vi "iPSread.vi"(8 "error in (no error)":errorcluster, 10 "iPSreadCtrl":T1=enum."Switch Heater Temp", 11 "VISA resource name":refnum<visa-resource-name>) -> (0 "error out":errorcluster, 1 "read buffer":string, 2 "number":dbl, 3 "VISA resource name out":refnum<visa-resource-name>)   [LabVIEW 2021]
uses:
  controls/iPSreadCtrl.ctl
  <vilib>/regexp/Match Regular Expression.xnode
panel:
  out "after match":string
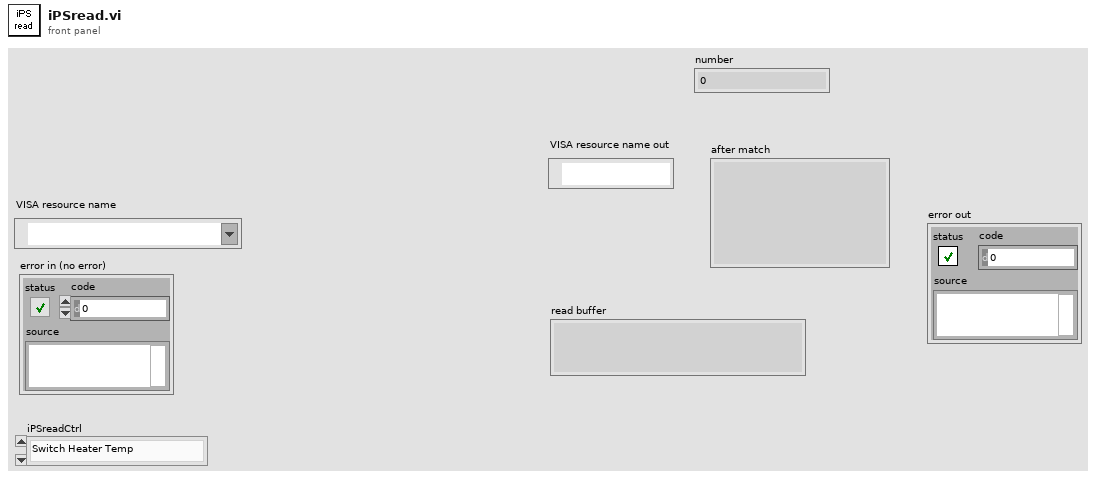
[diagram p1: front panel]
types:
  T1 = typedef "iPSreadCtrl.ctl" = enum16{"OutputField", "MagnetField", "Switch Heater Temp", "Field Rate", "Magnet Temp", "OutputVoltage"}
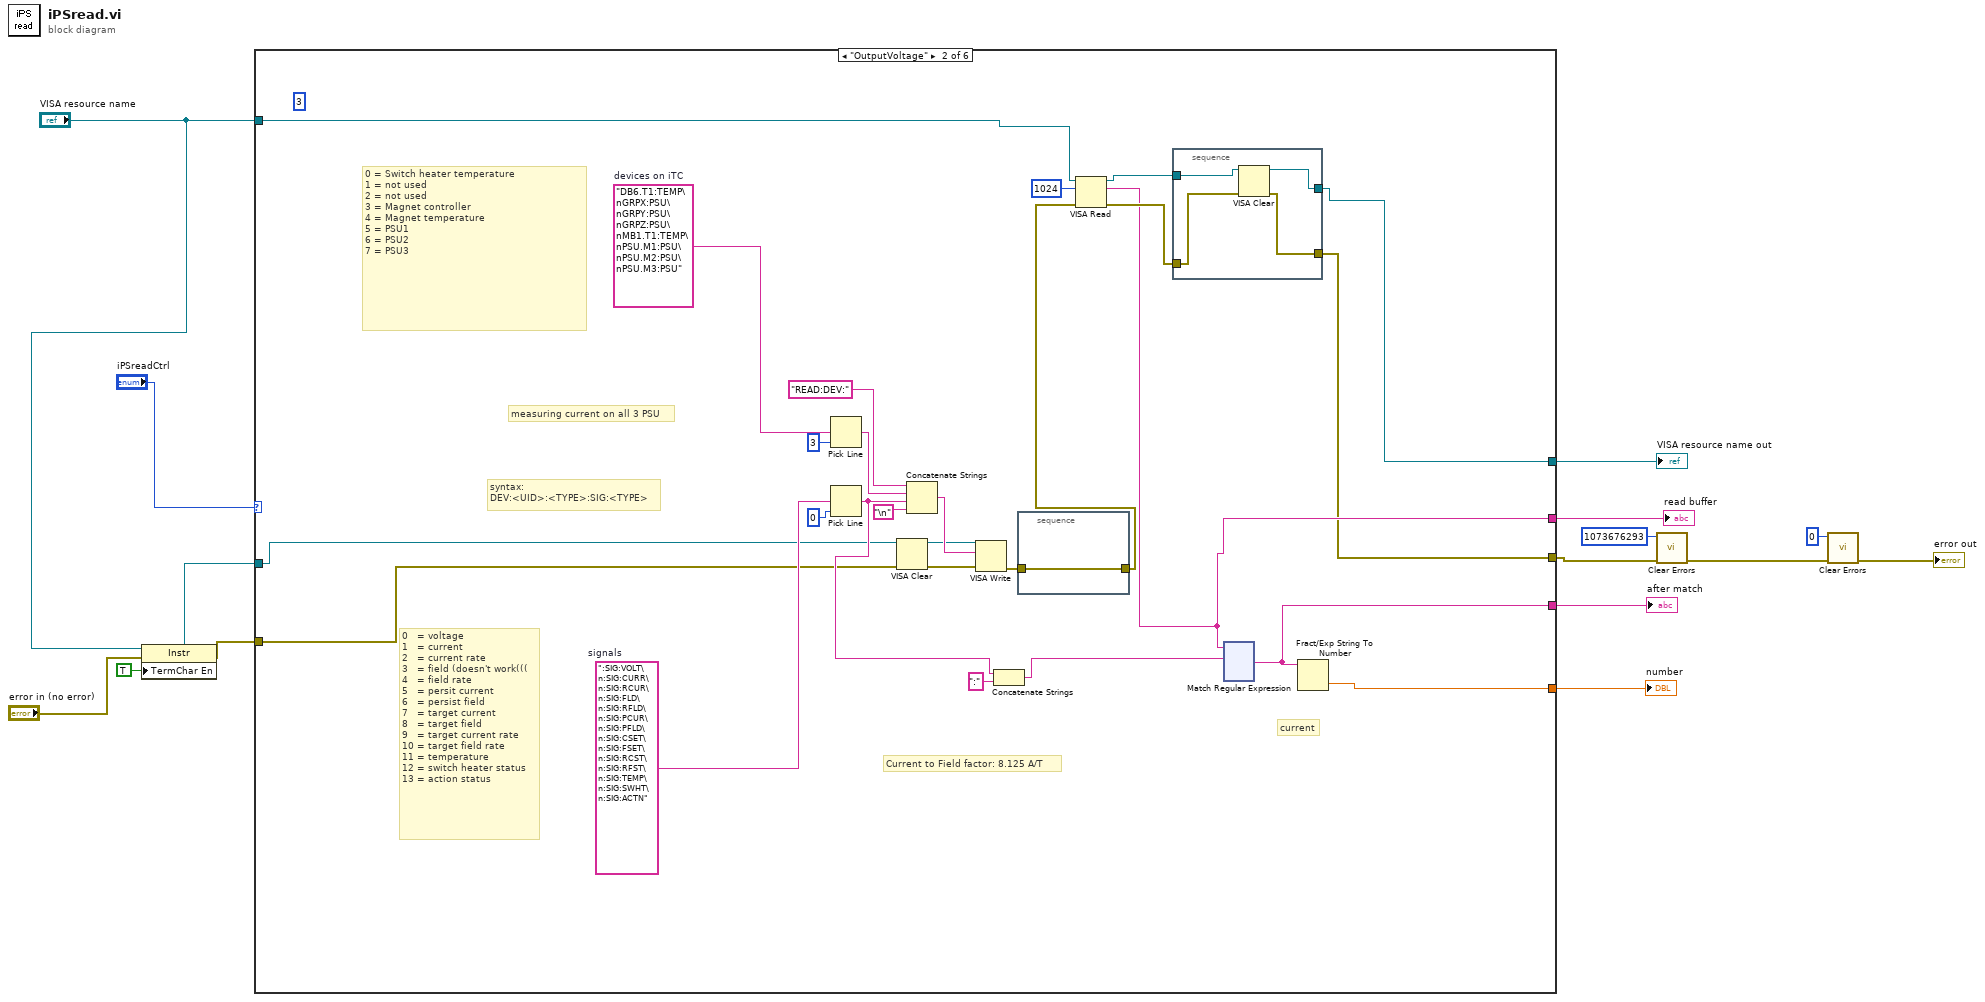
[diagram p0: block diagram]
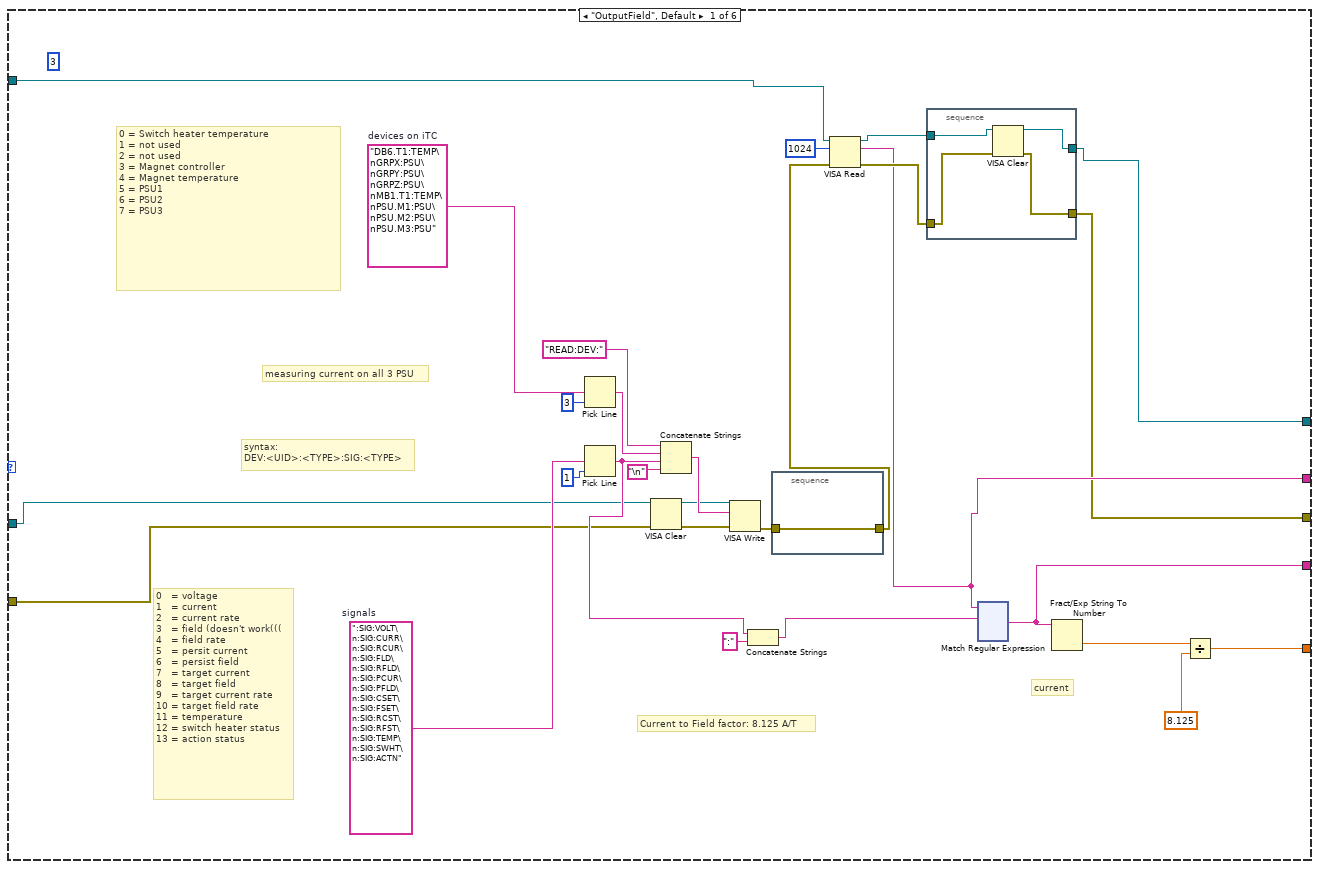
[diagram p2: hidden frame]
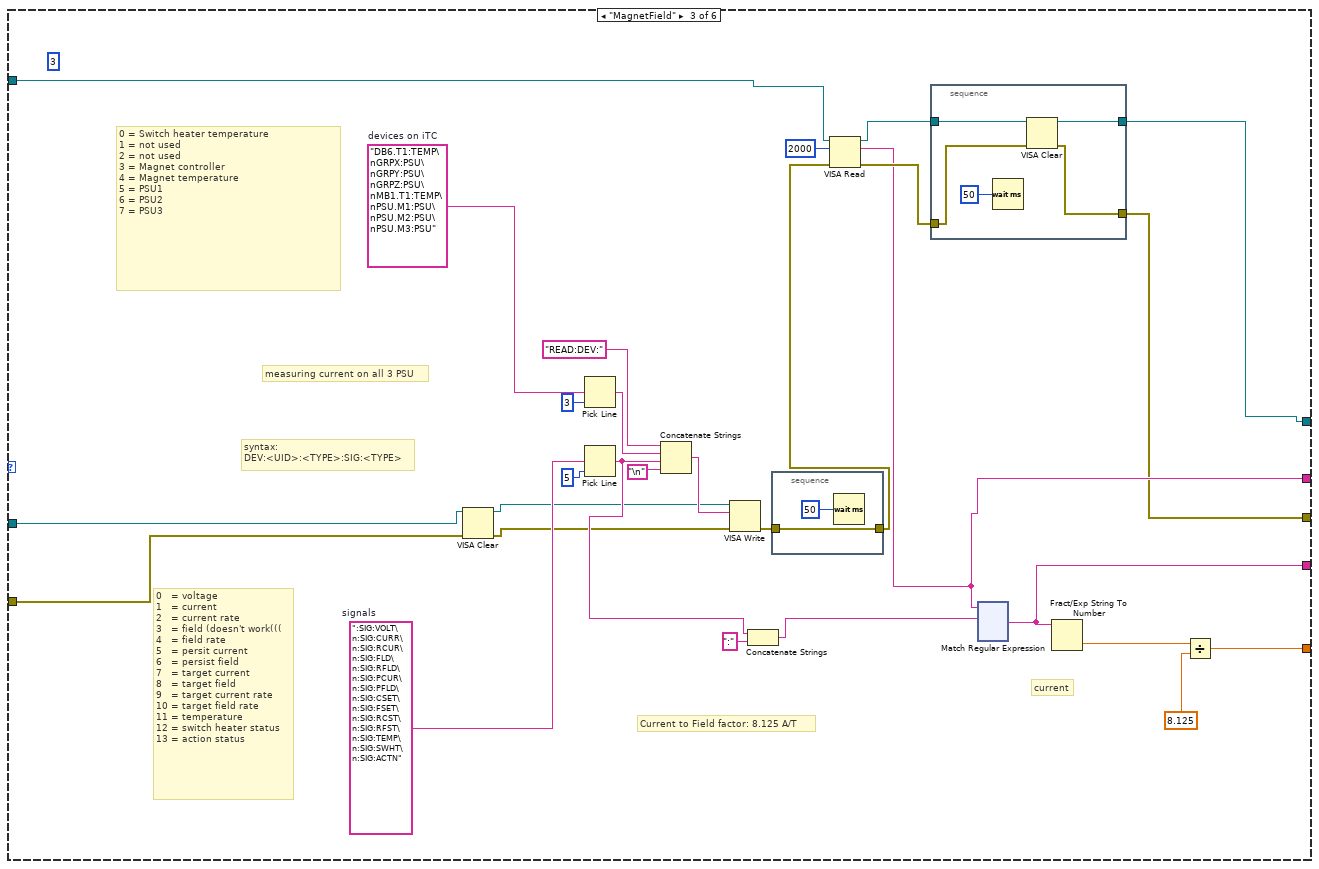
[diagram p3: hidden frame]
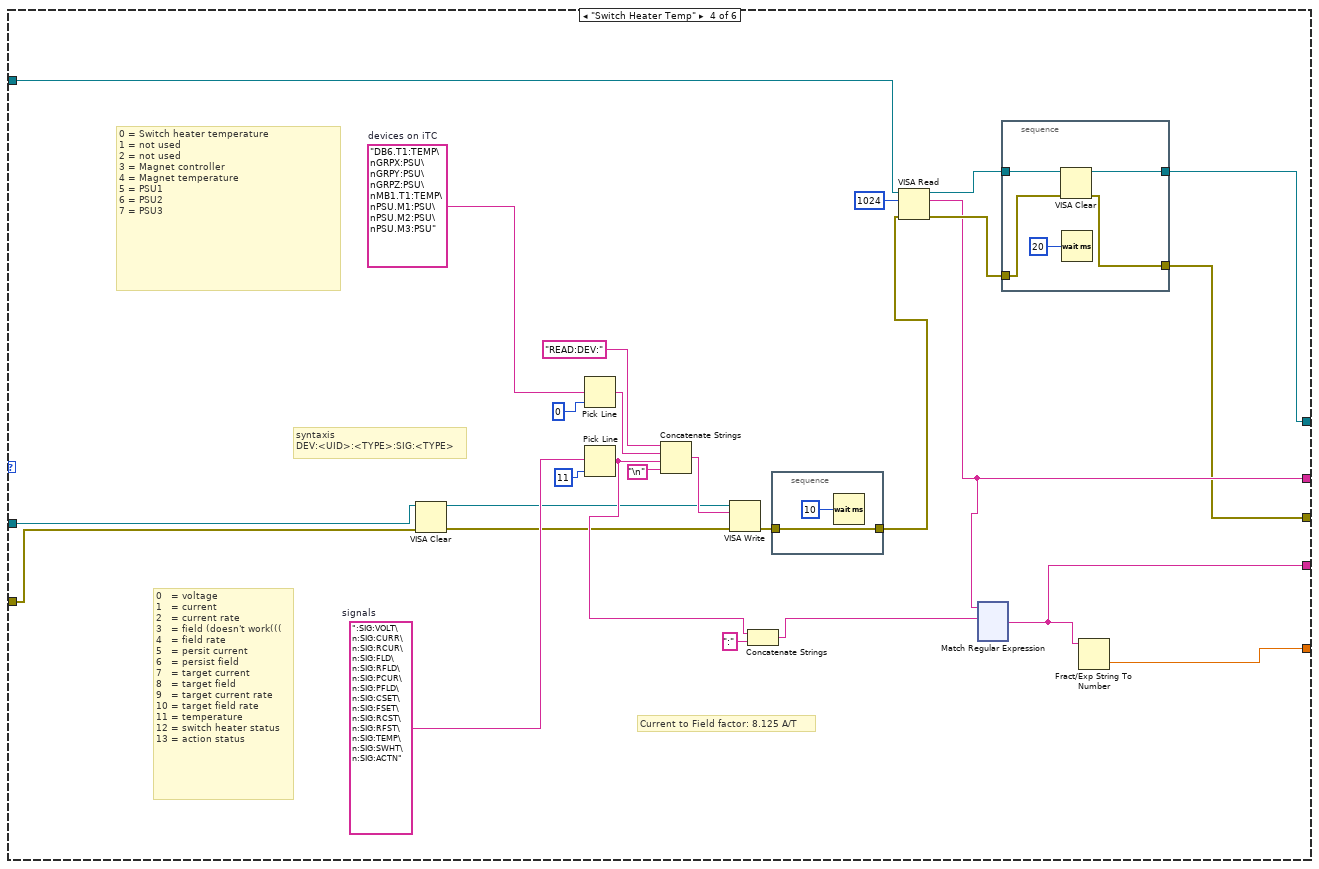
[diagram p4: hidden frame]
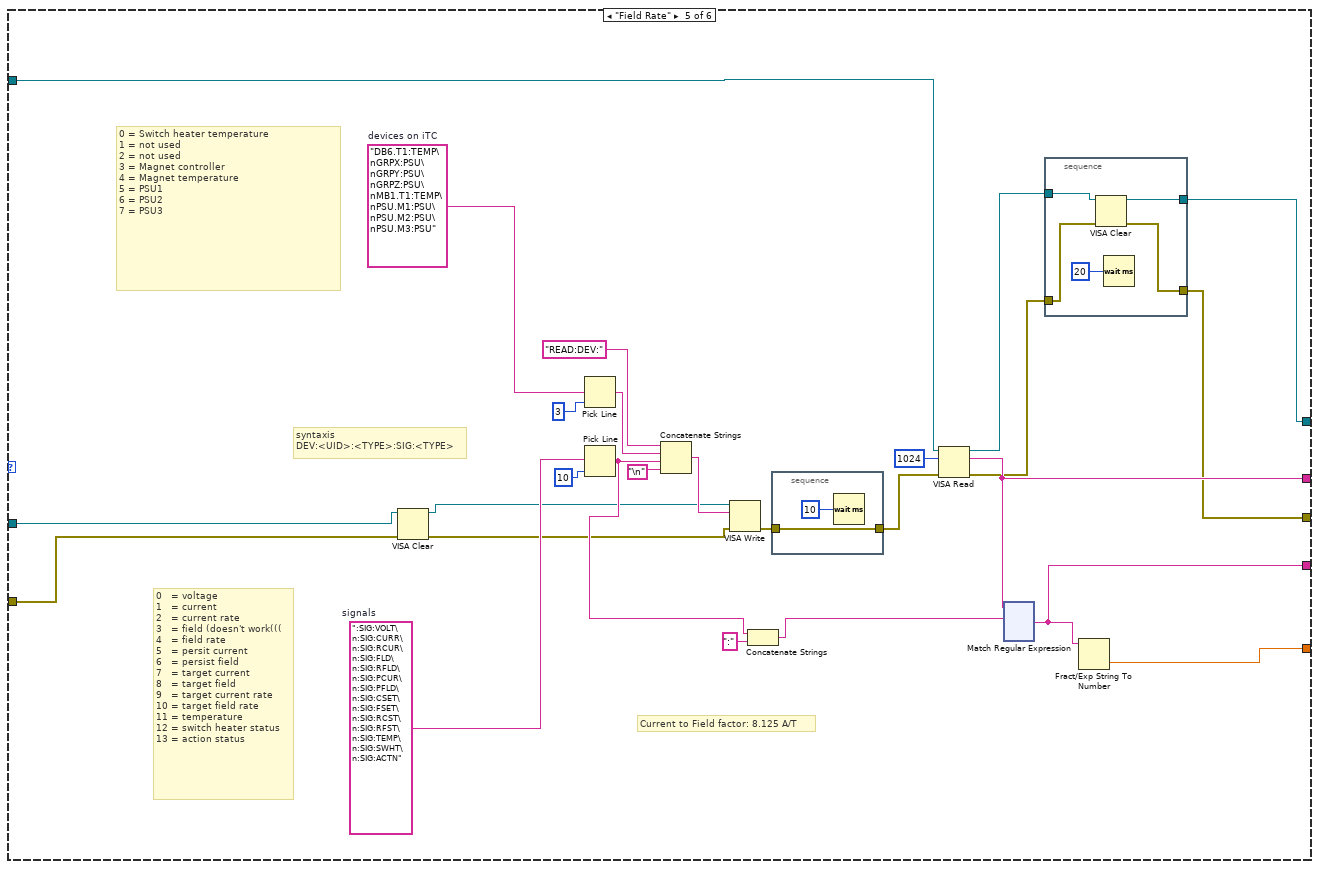
[diagram p5: hidden frame]
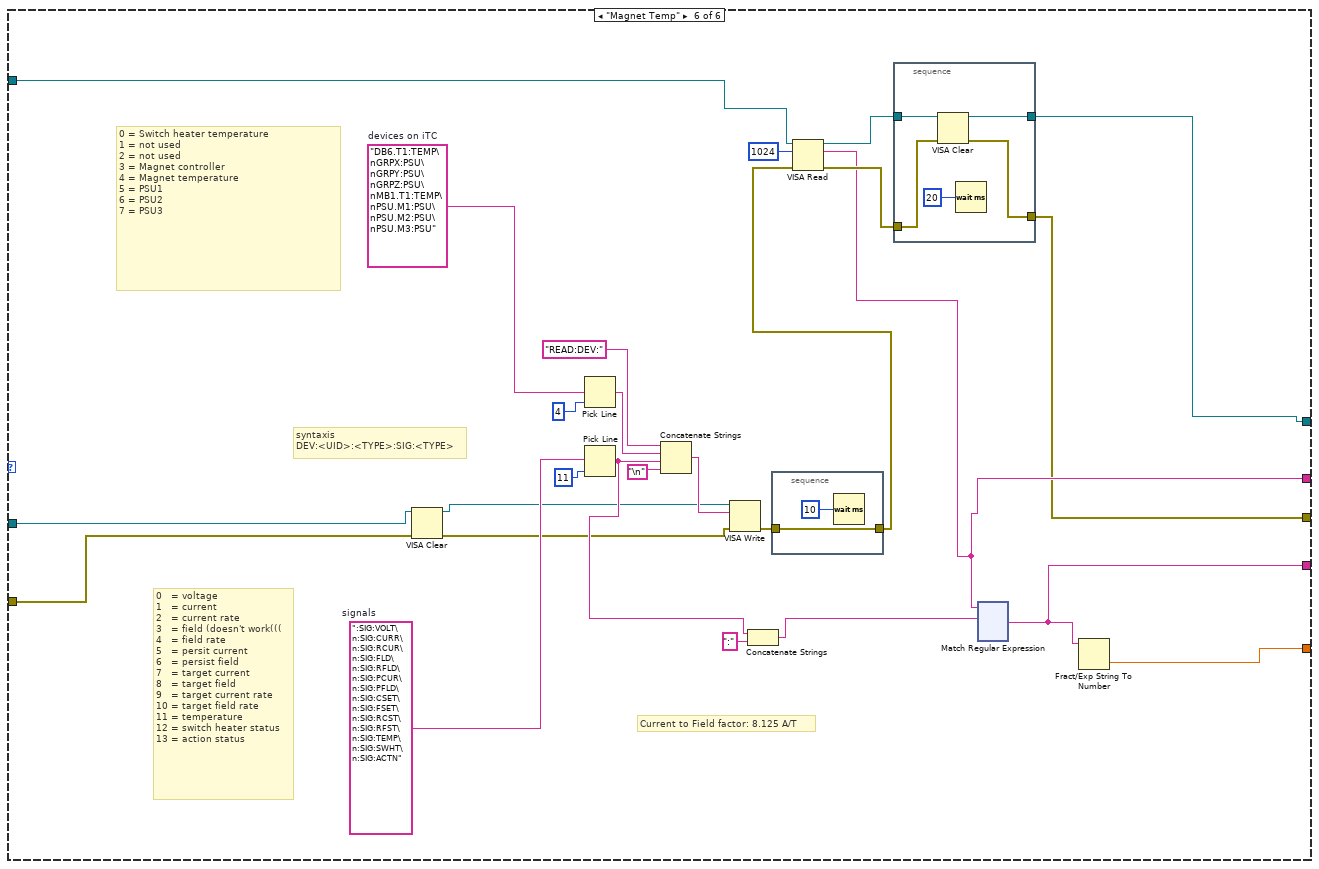
[diagram p6: hidden frame]
diagram:
  n1 = property class="Instr"(reference="VISA resource name", error in="error in (no error)", "TermChar En"=TRUE ("Message Based Settings:Termination Character Enable")) -> (reference out=w9:refnum<visa-resource-name>, error out=w7:errorcluster)
  n2 = case shown="\"OutputVoltage\"" "iPSreadCtrl" {
    tunnel: "VISA resource name" -> [w22 w173 w320 w472 w622 w775]
    tunnel: [w23 w174 w321 w473 w623 w772] -> w5
    tunnel: [w16 w167 w314 w467 w616 w767] -> w15
    tunnel: [w24 w175 w322 w475 w626 w773] -> w14
    tunnel: [w43 w191 w341 w481 w631 w781] -> w13
    tunnel: [w41 w166 w339 w480 w630 w780] -> w12
    tunnel: w7 -> [w20 w171 w316 w468 w620 w768]
    tunnel: w9 -> [w21 w172 w317 w469 w621 w769]
    frame "OutputField", Default {
      w35 = ":SIG:VOLT\n:SIG:CURR\n:SIG:RCUR\n:SIG:FLD\n:SIG:RFLD\n:SIG:PCUR\n:SIG:PFLD\n:SIG:CSET\n:SIG:FSET\n:SIG:RCST\n:SIG:RFST\n:SIG:TEMP\n:SIG:SWHT\n:SIG:ACTN"  # signals
      w40 = "DB6.T1:TEMP\nGRPX:PSU\nGRPY:PSU\nGRPZ:PSU\nMB1.T1:TEMP\nPSU.M1:PSU\nPSU.M2:PSU\nPSU.M3:PSU"  # devices on iTC
      (unwired) 3
      # "current"
      # "measuring current on all 3 PSU"
      # "Current to Field factor: 8.125 A/T"
      # "0 = Switch heater temperature\n1 = not used\n2 = not used\n3 = Magnet controller \n4 = Magnet temperature\n5 = PSU1 \n6 = PSU2\n7 = PSU3"
      # "0   = voltage\n1   = current\n2   = current rate\n3   = field (doesn't work(((\n4   = field rate\n5   = persit current\n6   = persist field\n7   = target current\n8   = target field\n9   = target current rate\n10 = target field rate \n11 = temperature\n12 = switch heater status\n13 = action status"
      # "syntax:\nDEV:<UID>:<TYPE>:SIG:<TYPE>"
      n3 = Pick Line(multi-line string=w40, line index=3) -> (output string=w37:string)  [unwired: 1 in]
      n4 = Pick Line(multi-line string=w35, line index=1) -> (output string=w33:string)  [unwired: 1 in]
      n5 = VISA Clear(VISA resource name=w21, error in (no error)=w20) -> (VISA resource name out=w19:refnum<visa-resource-name>, error out=w18:errorcluster)
      n6 = Concatenate Strings("READ:DEV:" ("write buffer"), w37, w33, "\n") -> (w31:string)
      n7 = VISA Write(VISA resource name=w19, write buffer=w31, error in (no error)=w18) -> (error out=w39:errorcluster)  [unwired: 2 out]
      n8 = Concatenate Strings(w33, ":" ("string")) -> (w32:string)
      n9 = stacked-sequence {
        tunnel: w39 -> [w165]
        tunnel: [w165] -> w25
        frame #0 {
        }
      }
      n10 = VISA Read(VISA resource name=w22, byte count=u32 1024, error in (no error)=w25) -> (VISA resource name out=w17:refnum<visa-resource-name>, read buffer=w24:string, error out=w26:errorcluster)  [unwired: 1 out]
      n11 = stacked-sequence {
        tunnel: [w46] -> w23
        tunnel: w26 -> [w45]
        tunnel: w17 -> [w44]
        tunnel: [w47] -> w16
        frame #0 {
          n12 = VISA Clear(VISA resource name=w44, error in (no error)=w45) -> (VISA resource name out=w47:refnum<visa-resource-name>, error out=w46:errorcluster)
        }
      }
      n13 = xnode "Match Regular Expression"("input string"=w24, "regular expression"=w32) -> ("after match"=w43:string)  [unwired: 4 in, 4 out]
      n14 = Fract/Exp String To Number(string=w43) -> (number=w28:dbl)  [unwired: 3 in, 1 out]
      n15 = Divide(x=w28, y=8.125) -> (x/y=w41:dbl)
    }
    frame "OutputVoltage" {
      w185 = ":SIG:VOLT\n:SIG:CURR\n:SIG:RCUR\n:SIG:FLD\n:SIG:RFLD\n:SIG:PCUR\n:SIG:PFLD\n:SIG:CSET\n:SIG:FSET\n:SIG:RCST\n:SIG:RFST\n:SIG:TEMP\n:SIG:SWHT\n:SIG:ACTN"  # signals
      w190 = "DB6.T1:TEMP\nGRPX:PSU\nGRPY:PSU\nGRPZ:PSU\nMB1.T1:TEMP\nPSU.M1:PSU\nPSU.M2:PSU\nPSU.M3:PSU"  # devices on iTC
      (unwired) 3
      # "current"
      # "measuring current on all 3 PSU"
      # "Current to Field factor: 8.125 A/T"
      # "0 = Switch heater temperature\n1 = not used\n2 = not used\n3 = Magnet controller \n4 = Magnet temperature\n5 = PSU1 \n6 = PSU2\n7 = PSU3"
      # "0   = voltage\n1   = current\n2   = current rate\n3   = field (doesn't work(((\n4   = field rate\n5   = persit current\n6   = persist field\n7   = target current\n8   = target field\n9   = target current rate\n10 = target field rate \n11 = temperature\n12 = switch heater status\n13 = action status"
      # "syntax:\nDEV:<UID>:<TYPE>:SIG:<TYPE>"
      n16 = Pick Line(multi-line string=w190, line index=3) -> (output string=w187:string)  [unwired: 1 in]
      n17 = Pick Line(multi-line string=w185, line index=0) -> (output string=w183:string)  [unwired: 1 in]
      n18 = VISA Clear(VISA resource name=w172, error in (no error)=w171) -> (VISA resource name out=w170:refnum<visa-resource-name>, error out=w169:errorcluster)
      n19 = Concatenate Strings("READ:DEV:" ("write buffer"), w187, w183, "\n") -> (w181:string)
      n20 = VISA Write(VISA resource name=w170, write buffer=w181, error in (no error)=w169) -> (error out=w189:errorcluster)  [unwired: 2 out]
      n21 = Concatenate Strings(w183, ":" ("string")) -> (w182:string)
      n22 = stacked-sequence {
        tunnel: w189 -> [w313]
        tunnel: [w313] -> w176
        frame #0 {
        }
      }
      n23 = VISA Read(VISA resource name=w173, byte count=u32 1024, error in (no error)=w176) -> (VISA resource name out=w168:refnum<visa-resource-name>, read buffer=w175:string, error out=w177:errorcluster)  [unwired: 1 out]
      n24 = stacked-sequence {
        tunnel: [w194] -> w174
        tunnel: w177 -> [w193]
        tunnel: w168 -> [w192]
        tunnel: [w195] -> w167
        frame #0 {
          n25 = VISA Clear(VISA resource name=w192, error in (no error)=w193) -> (VISA resource name out=w195:refnum<visa-resource-name>, error out=w194:errorcluster)
        }
      }
      n26 = xnode "Match Regular Expression"("input string"=w175, "regular expression"=w182) -> ("after match"=w191:string)  [unwired: 4 in, 4 out]
      n27 = Fract/Exp String To Number(string=w191) -> (number=w166:dbl)  [unwired: 3 in, 1 out]
    }
    frame "MagnetField" {
      w333 = ":SIG:VOLT\n:SIG:CURR\n:SIG:RCUR\n:SIG:FLD\n:SIG:RFLD\n:SIG:PCUR\n:SIG:PFLD\n:SIG:CSET\n:SIG:FSET\n:SIG:RCST\n:SIG:RFST\n:SIG:TEMP\n:SIG:SWHT\n:SIG:ACTN"  # signals
      w338 = "DB6.T1:TEMP\nGRPX:PSU\nGRPY:PSU\nGRPZ:PSU\nMB1.T1:TEMP\nPSU.M1:PSU\nPSU.M2:PSU\nPSU.M3:PSU"  # devices on iTC
      (unwired) 3
      # "current"
      # "measuring current on all 3 PSU"
      # "Current to Field factor: 8.125 A/T"
      # "0 = Switch heater temperature\n1 = not used\n2 = not used\n3 = Magnet controller \n4 = Magnet temperature\n5 = PSU1 \n6 = PSU2\n7 = PSU3"
      # "0   = voltage\n1   = current\n2   = current rate\n3   = field (doesn't work(((\n4   = field rate\n5   = persit current\n6   = persist field\n7   = target current\n8   = target field\n9   = target current rate\n10 = target field rate \n11 = temperature\n12 = switch heater status\n13 = action status"
      # "syntax:\nDEV:<UID>:<TYPE>:SIG:<TYPE>"
      n28 = VISA Clear(VISA resource name=w317, error in (no error)=w316) -> (VISA resource name out=w319:refnum<visa-resource-name>, error out=w318:errorcluster)
      n29 = Pick Line(multi-line string=w338, line index=3) -> (output string=w335:string)  [unwired: 1 in]
      n30 = Pick Line(multi-line string=w333, line index=5) -> (output string=w331:string)  [unwired: 1 in]
      n31 = Concatenate Strings("READ:DEV:" ("write buffer"), w335, w331, "\n") -> (w329:string)
      n32 = VISA Write(VISA resource name=w319, write buffer=w329, error in (no error)=w318) -> (error out=w337:errorcluster)  [unwired: 2 out]
      n33 = Concatenate Strings(w331, ":" ("string")) -> (w330:string)
      n34 = stacked-sequence {
        tunnel: w337 -> [w465]
        tunnel: [w465] -> w323
        frame #0 {
          n35 = Wait (ms)(milliseconds to wait=u32 50) -> ()  [unwired: 1 out]
        }
      }
      n36 = VISA Read(VISA resource name=w320, byte count=u32 2000, error in (no error)=w323) -> (VISA resource name out=w315:refnum<visa-resource-name>, read buffer=w322:string, error out=w324:errorcluster)  [unwired: 1 out]
      n37 = stacked-sequence {
        tunnel: [w343] -> w321
        tunnel: w324 -> [w342]
        tunnel: w315 -> [w345]
        tunnel: [w344] -> w314
        frame #0 {
          n38 = Wait (ms)(milliseconds to wait=u32 50) -> ()  [unwired: 1 out]
          n39 = VISA Clear(VISA resource name=w345, error in (no error)=w342) -> (VISA resource name out=w344:refnum<visa-resource-name>, error out=w343:errorcluster)
        }
      }
      n40 = xnode "Match Regular Expression"("input string"=w322, "regular expression"=w330) -> ("after match"=w341:string)  [unwired: 4 in, 4 out]
      n41 = Fract/Exp String To Number(string=w341) -> (number=w326:dbl)  [unwired: 3 in, 1 out]
      n42 = Divide(x=w326, y=8.125) -> (x/y=w339:dbl)
    }
    frame "Switch Heater Temp" {
      w486 = ":SIG:VOLT\n:SIG:CURR\n:SIG:RCUR\n:SIG:FLD\n:SIG:RFLD\n:SIG:PCUR\n:SIG:PFLD\n:SIG:CSET\n:SIG:FSET\n:SIG:RCST\n:SIG:RFST\n:SIG:TEMP\n:SIG:SWHT\n:SIG:ACTN"  # signals
      w491 = "DB6.T1:TEMP\nGRPX:PSU\nGRPY:PSU\nGRPZ:PSU\nMB1.T1:TEMP\nPSU.M1:PSU\nPSU.M2:PSU\nPSU.M3:PSU"  # devices on iTC
      # "Current to Field factor: 8.125 A/T"
      # "0 = Switch heater temperature\n1 = not used\n2 = not used\n3 = Magnet controller \n4 = Magnet temperature\n5 = PSU1 \n6 = PSU2\n7 = PSU3"
      # "0   = voltage\n1   = current\n2   = current rate\n3   = field (doesn't work(((\n4   = field rate\n5   = persit current\n6   = persist field\n7   = target current\n8   = target field\n9   = target current rate\n10 = target field rate \n11 = temperature\n12 = switch heater status\n13 = action status"
      # "syntaxis\nDEV:<UID>:<TYPE>:SIG:<TYPE>"
      n43 = VISA Clear(VISA resource name=w469, error in (no error)=w468) -> (VISA resource name out=w471:refnum<visa-resource-name>, error out=w470:errorcluster)
      n44 = Pick Line(multi-line string=w491, line index=0) -> (output string=w488:string)  [unwired: 1 in]
      n45 = Pick Line(multi-line string=w486, line index=11) -> (output string=w484:string)  [unwired: 1 in]
      n46 = Concatenate Strings("READ:DEV:" ("write buffer"), w488, w484, "\n") -> (w482:string)
      n47 = VISA Write(VISA resource name=w471, write buffer=w482, error in (no error)=w470) -> (error out=w490:errorcluster)  [unwired: 2 out]
      n48 = Concatenate Strings(w484, ":" ("string")) -> (w483:string)
      n49 = stacked-sequence {
        tunnel: w490 -> [w615]
        tunnel: [w615] -> w474
        frame #0 {
          n50 = Wait (ms)(milliseconds to wait=u32 10) -> ()  [unwired: 1 out]
        }
      }
      n51 = VISA Read(VISA resource name=w472, byte count=u32 1024, error in (no error)=w474) -> (VISA resource name out=w466:refnum<visa-resource-name>, read buffer=w475:string, error out=w476:errorcluster)  [unwired: 1 out]
      n52 = xnode "Match Regular Expression"("input string"=w475, "regular expression"=w483) -> ("after match"=w481:string)  [unwired: 4 in, 4 out]
      n53 = stacked-sequence {
        tunnel: [w495] -> w473
        tunnel: w476 -> [w494]
        tunnel: [w493] -> w467
        tunnel: w466 -> [w492]
        frame #0 {
          n54 = VISA Clear(VISA resource name=w492, error in (no error)=w494) -> (VISA resource name out=w493:refnum<visa-resource-name>, error out=w495:errorcluster)
          n55 = Wait (ms)(milliseconds to wait=u32 20) -> ()  [unwired: 1 out]
        }
      }
      n56 = Fract/Exp String To Number(string=w481) -> (number=w480:dbl)  [unwired: 3 in, 1 out]
    }
    frame "Field Rate" {
      w636 = ":SIG:VOLT\n:SIG:CURR\n:SIG:RCUR\n:SIG:FLD\n:SIG:RFLD\n:SIG:PCUR\n:SIG:PFLD\n:SIG:CSET\n:SIG:FSET\n:SIG:RCST\n:SIG:RFST\n:SIG:TEMP\n:SIG:SWHT\n:SIG:ACTN"  # signals
      w641 = "DB6.T1:TEMP\nGRPX:PSU\nGRPY:PSU\nGRPZ:PSU\nMB1.T1:TEMP\nPSU.M1:PSU\nPSU.M2:PSU\nPSU.M3:PSU"  # devices on iTC
      # "Current to Field factor: 8.125 A/T"
      # "0 = Switch heater temperature\n1 = not used\n2 = not used\n3 = Magnet controller \n4 = Magnet temperature\n5 = PSU1 \n6 = PSU2\n7 = PSU3"
      # "0   = voltage\n1   = current\n2   = current rate\n3   = field (doesn't work(((\n4   = field rate\n5   = persit current\n6   = persist field\n7   = target current\n8   = target field\n9   = target current rate\n10 = target field rate \n11 = temperature\n12 = switch heater status\n13 = action status"
      # "syntaxis\nDEV:<UID>:<TYPE>:SIG:<TYPE>"
      n57 = VISA Clear(VISA resource name=w621, error in (no error)=w620) -> (VISA resource name out=w619:refnum<visa-resource-name>, error out=w618:errorcluster)
      n58 = Pick Line(multi-line string=w641, line index=3) -> (output string=w638:string)  [unwired: 1 in]
      n59 = Pick Line(multi-line string=w636, line index=10) -> (output string=w634:string)  [unwired: 1 in]
      n60 = Concatenate Strings("READ:DEV:" ("write buffer"), w638, w634, "\n") -> (w632:string)
      n61 = VISA Write(VISA resource name=w619, write buffer=w632, error in (no error)=w618) -> (error out=w640:errorcluster)  [unwired: 2 out]
      n62 = Concatenate Strings(w634, ":" ("string")) -> (w633:string)
      n63 = stacked-sequence {
        tunnel: w640 -> [w765]
        tunnel: [w765] -> w625
        frame #0 {
          n64 = Wait (ms)(milliseconds to wait=u32 10) -> ()  [unwired: 1 out]
        }
      }
      n65 = VISA Read(VISA resource name=w622, byte count=u32 1024, error in (no error)=w625) -> (VISA resource name out=w617:refnum<visa-resource-name>, read buffer=w626:string, error out=w624:errorcluster)  [unwired: 1 out]
      n66 = xnode "Match Regular Expression"("input string"=w626, "regular expression"=w633) -> ("after match"=w631:string)  [unwired: 4 in, 4 out]
      n67 = stacked-sequence {
        tunnel: [w645] -> w623
        tunnel: w624 -> [w644]
        tunnel: w617 -> [w643]
        tunnel: [w642] -> w616
        frame #0 {
          n68 = VISA Clear(VISA resource name=w643, error in (no error)=w644) -> (VISA resource name out=w642:refnum<visa-resource-name>, error out=w645:errorcluster)
          n69 = Wait (ms)(milliseconds to wait=u32 20) -> ()  [unwired: 1 out]
        }
      }
      n70 = Fract/Exp String To Number(string=w631) -> (number=w630:dbl)  [unwired: 3 in, 1 out]
    }
    frame "Magnet Temp" {
      w786 = ":SIG:VOLT\n:SIG:CURR\n:SIG:RCUR\n:SIG:FLD\n:SIG:RFLD\n:SIG:PCUR\n:SIG:PFLD\n:SIG:CSET\n:SIG:FSET\n:SIG:RCST\n:SIG:RFST\n:SIG:TEMP\n:SIG:SWHT\n:SIG:ACTN"  # signals
      w791 = "DB6.T1:TEMP\nGRPX:PSU\nGRPY:PSU\nGRPZ:PSU\nMB1.T1:TEMP\nPSU.M1:PSU\nPSU.M2:PSU\nPSU.M3:PSU"  # devices on iTC
      # "Current to Field factor: 8.125 A/T"
      # "0 = Switch heater temperature\n1 = not used\n2 = not used\n3 = Magnet controller \n4 = Magnet temperature\n5 = PSU1 \n6 = PSU2\n7 = PSU3"
      # "0   = voltage\n1   = current\n2   = current rate\n3   = field (doesn't work(((\n4   = field rate\n5   = persit current\n6   = persist field\n7   = target current\n8   = target field\n9   = target current rate\n10 = target field rate \n11 = temperature\n12 = switch heater status\n13 = action status"
      # "syntaxis\nDEV:<UID>:<TYPE>:SIG:<TYPE>"
      n71 = VISA Clear(VISA resource name=w769, error in (no error)=w768) -> (VISA resource name out=w771:refnum<visa-resource-name>, error out=w770:errorcluster)
      n72 = Pick Line(multi-line string=w791, line index=4) -> (output string=w788:string)  [unwired: 1 in]
      n73 = Pick Line(multi-line string=w786, line index=11) -> (output string=w784:string)  [unwired: 1 in]
      n74 = Concatenate Strings("READ:DEV:" ("write buffer"), w788, w784, "\n") -> (w782:string)
      n75 = VISA Write(VISA resource name=w771, write buffer=w782, error in (no error)=w770) -> (error out=w790:errorcluster)  [unwired: 2 out]
      n76 = Concatenate Strings(w784, ":" ("string")) -> (w783:string)
      n77 = stacked-sequence {
        tunnel: w790 -> [w915]
        tunnel: [w915] -> w774
        frame #0 {
          n78 = Wait (ms)(milliseconds to wait=u32 10) -> ()  [unwired: 1 out]
        }
      }
      n79 = VISA Read(VISA resource name=w775, byte count=u32 1024, error in (no error)=w774) -> (VISA resource name out=w766:refnum<visa-resource-name>, read buffer=w773:string, error out=w776:errorcluster)  [unwired: 1 out]
      n80 = stacked-sequence {
        tunnel: [w795] -> w772
        tunnel: w776 -> [w794]
        tunnel: [w793] -> w767
        tunnel: w766 -> [w792]
        frame #0 {
          n81 = VISA Clear(VISA resource name=w792, error in (no error)=w794) -> (VISA resource name out=w793:refnum<visa-resource-name>, error out=w795:errorcluster)
          n82 = Wait (ms)(milliseconds to wait=u32 20) -> ()  [unwired: 1 out]
        }
      }
      n83 = xnode "Match Regular Expression"("input string"=w773, "regular expression"=w783) -> ("after match"=w781:string)  [unwired: 4 in, 4 out]
      n84 = Fract/Exp String To Number(string=w781) -> (number=w780:dbl)  [unwired: 3 in, 1 out]
    }
  }
  "read buffer" <- w14
  "VISA resource name out" <- w15
  "after match" <- w13
  "number" <- w12
  n85 = call <vilib>:"Clear Errors.vi"("error in (no error)"=w5, "specific error code to clear (0: all)"=1073676293) -> ("error out"=w3:errorcluster)  [unwired: 4 in, 1 out]
  n86 = call <vilib>:"Clear Errors.vi"("error in (no error)"=w3, "specific error code to clear (0: all)"=0) -> ("error out"=→"error out":errorcluster)  [unwired: 4 in, 1 out]
